vi "read_serie_monitor  (1).vi"() -> ()   [LabVIEW 2012]
uses:
  <vilib>/Instr/_visa.llb/VISA Configure Serial Port (Instr).vi
panel:
  in  "baud rate":u32=9600
  in  "offset":i32
  out "Data":string
  in  "COM Port":refnum<visa-resource-name>
  in  "read":bool
  in  "stop":bool
  out "Signal":i32(graph)
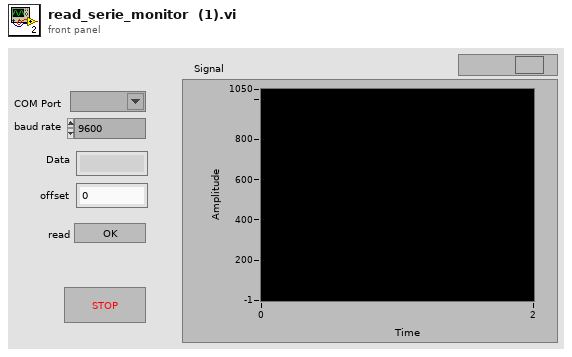
[diagram p1: front panel]
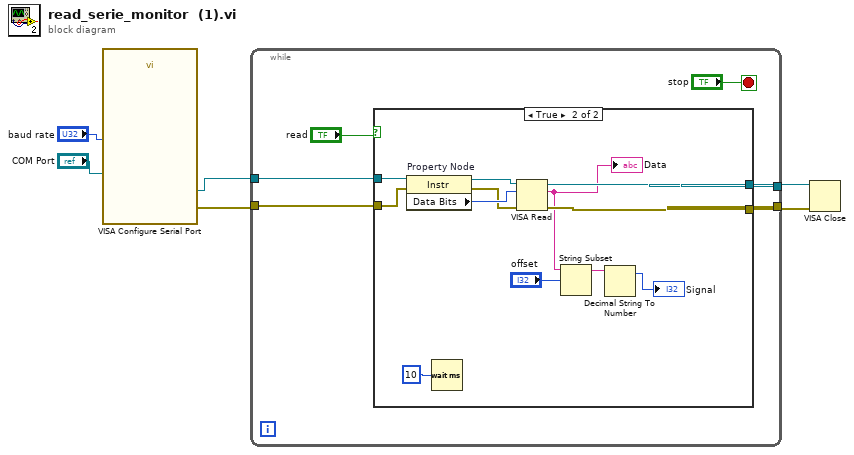
[diagram p0: block diagram]
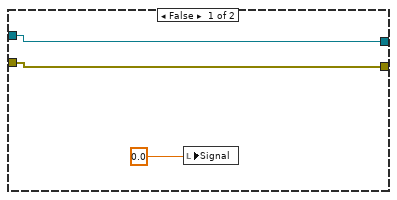
[diagram p2: hidden frame]
diagram:
  n1 = call-poly "VISA Configure Serial Port"("VISA resource name"="COM Port", "baud rate (9600)"="baud rate") -> ("VISA resource name out"=w3:refnum<visa-resource-name>, "error out"=w2:errorcluster)  [unwired: 12 in]
  n2 = while {
    tunnel: [w12] -> w5
    tunnel: [w11] -> w4
    tunnel: w3 -> [w10]
    tunnel: w2 -> [w9]
    stop <- "stop" stop-if-true
    n3 = case shown="True" "read" {
      tunnel: [w14 w27] -> w12
      tunnel: [w15 w24] -> w11
      tunnel: w10 -> [w14 w22]
      tunnel: w9 -> [w15 w21]
      frame False {
        n4 = local write "Signal"(0.0 ("Signal")) -> ()
      }
      frame True {
        n5 = property on="Property Node" class="Instr"(reference=w22, error in=w21) -> (reference out=w23:refnum<visa-resource-name>, error out=w25:errorcluster, "Data Bits"=w26:u16)
        n6 = Wait (ms)(milliseconds to wait=u32 10) -> ()  [unwired: 1 out]
        n7 = VISA Read(VISA resource name=w23, byte count=w26, error in (no error)=w25) -> (VISA resource name out=w27:refnum<visa-resource-name>, read buffer=w18:string, error out=w24:errorcluster)  [unwired: 1 out]
        "Data" <- w18
        n8 = String Subset(string=w18, offset (0)="offset") -> (substring=w20:string)  [unwired: 1 in]
        n9 = Decimal String To Number(string=w20) -> (offset past number=→"Signal":i32)  [unwired: 2 in, 1 out]
      }
    }
  }
  n10 = VISA Close(VISA resource name=w5, error in (no error)=w4) -> ()  [unwired: 1 out]
